vi "VI Tree.vi"   [LabVIEW 2021, in "Lake Shore 336.lvlib"]
doc: "This is the instrument driver for the Lake Shore Model 336 Temperature Controller. The VI Tree displays all the user-callable VIs of the instrument driver in an organized table."
uses:
  <instrlib>/Lake Shore 336/Lake Shore 336.lvlib
  <instrlib>/Lake Shore 336/Public/Data/Sensor Data (Single Reading).vi
panel:
  # "(c) 2009 Lake Shore Cryotronics Inc.  ALL RIGHTS RESERVED."
  # "SEE DIAGRAM\nFOR VI TREE."
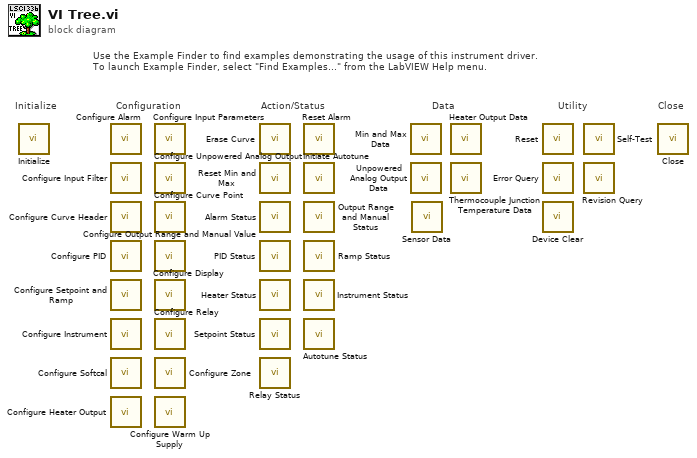
[diagram p0: block diagram]
diagram:
  # "Configuration"
  # "Utility"
  # "Data"
  # "Action/Status"
  # "Close"
  # "Initialize"
  # "Use the Example Finder to find examples demonstrating the usage of this instrument driver.\nTo launch Example Finder, select \"Find Examples...\" from the LabVIEW Help menu."
  n1 = call <instrlib>:"Initialize.vi"() -> ()  [unwired: 10 in, 2 out]
  n2 = call <instrlib>:"Configure Alarm.vi"() -> ()  [unwired: 14 in, 2 out]
  n3 = call <instrlib>:"Configure Input Filter.vi"() -> ()  [unwired: 14 in, 2 out]
  n4 = call <instrlib>:"Configure Curve Header.vi"() -> ()  [unwired: 14 in, 2 out]
  n5 = call <instrlib>:"Configure PID.vi"() -> ()  [unwired: 14 in, 2 out]
  n6 = call <instrlib>:"Configure Setpoint and Ramp.vi"() -> ()  [unwired: 14 in, 2 out]
  n7 = call <instrlib>:"Configure Instrument.vi"() -> ()  [unwired: 14 in, 2 out]
  n8 = call <instrlib>:"Configure Softcal.vi"() -> ()  [unwired: 14 in, 2 out]
  n9 = call <instrlib>:"Configure Heater Output.vi"() -> ()  [unwired: 14 in, 2 out]
  n10 = call <instrlib>:"Configure Input Parameters.vi"() -> ()  [unwired: 14 in, 2 out]
  n11 = call <instrlib>:"Configure Unpowered Analog Output.vi"() -> ()  [unwired: 14 in, 2 out]
  n12 = call <instrlib>:"Configure Curve Point.vi"() -> ()  [unwired: 14 in, 2 out]
  n13 = call <instrlib>:"Configure Output Range and Manual Value.vi"() -> ()  [unwired: 14 in, 2 out]
  n14 = call <instrlib>:"Configure Display.vi"() -> ()  [unwired: 14 in, 2 out]
  n15 = call <instrlib>:"Configure Relay.vi"() -> ()  [unwired: 14 in, 2 out]
  n16 = call <instrlib>:"Configure Zone.vi"() -> ()  [unwired: 14 in, 2 out]
  n17 = call <instrlib>:"Configure Warm Up Supply.vi"() -> ()  [unwired: 14 in, 2 out]
  n18 = call <instrlib>:"Erase Curve.vi"() -> ()  [unwired: 10 in, 2 out]
  n19 = call <instrlib>:"Reset Min and Max.vi"() -> ()  [unwired: 10 in, 2 out]
  n20 = call <instrlib>:"Alarm Status.vi"() -> ()  [unwired: 8 in, 4 out]
  n21 = call <instrlib>:"PID Status.vi"() -> ()  [unwired: 7 in, 5 out]
  n22 = call <instrlib>:"Heater Status.vi"() -> ()  [unwired: 9 in, 3 out]
  n23 = call <instrlib>:"Setpoint Status.vi"() -> ()  [unwired: 9 in, 3 out]
  n24 = call <instrlib>:"Relay Status.vi"() -> ()  [unwired: 9 in, 3 out]
  n25 = call <instrlib>:"Reset Alarm.vi"() -> ()  [unwired: 10 in, 2 out]
  n26 = call <instrlib>:"Initiate Autotune.vi"() -> ()  [unwired: 14 in, 2 out]
  n27 = call <instrlib>:"Output Range and Manual Status.vi"() -> ()  [unwired: 8 in, 4 out]
  n28 = call <instrlib>:"Ramp Status.vi"() -> ()  [unwired: 7 in, 5 out]
  n29 = call <instrlib>:"Instrument Status.vi"() -> ()  [unwired: 7 in, 5 out]
  n30 = call <instrlib>:"Autotune Status.vi"() -> ()  [unwired: 6 in, 6 out]
  n31 = call <instrlib>:"Min and Max Data.vi"() -> ()  [unwired: 8 in, 4 out]
  n32 = call <instrlib>:"Unpowered Analog Output Data.vi"() -> ()  [unwired: 9 in, 3 out]
  n33 = call-poly <instrlib>:"Sensor Data.vi"() -> ()  [unwired: 9 in, 3 out]
  n34 = call <instrlib>:"Heater Output Data.vi"() -> ()  [unwired: 9 in, 3 out]
  n35 = call <instrlib>:"Thermocouple Junction Temperature Data.vi"() -> ()  [unwired: 9 in, 3 out]
  n36 = call <instrlib>:"Reset.vi"() -> ()  [unwired: 10 in, 2 out]
  n37 = call <instrlib>:"Error Query.vi"() -> ()  [unwired: 9 in, 3 out]
  n38 = call <instrlib>:"Device Clear.vi"() -> ()  [unwired: 10 in, 2 out]
  n39 = call <instrlib>:"Self-Test.vi"() -> ()  [unwired: 8 in, 4 out]
  n40 = call <instrlib>:"Revision Query.vi"() -> ()  [unwired: 5 in, 7 out]
  n41 = call <instrlib>:"Close.vi"() -> ()  [unwired: 11 in, 1 out]
